vi "PurePursuit.vi"(0 "RobotNeededPathData":T1={"Path"=[], "MaxVel"=0.0, "MaxAccel"=0.0, "Backwards?"=FALSE, "PointSpacing"=0.0, "LookaheadDist"=0.0, "Speed/Curve"=1.8, "SlowDistanceAtEnd"=12.0, "SlowSpeed"=15.0, "MaxDeAccel"=0.0} {"SlowSpeed" format="%#_13g"; "SlowDistanceAtEnd" format="%#_13g"; "Speed/Curve" format="%#_13g"}, 1 "SensorData":T3={"LeftDistance"=0.0, "RightDistance"=0.0, "LeftVelocity"=78.75762159095939, "RightVelocity"=-76.3848555077329, "Angle"=-0.01, "Location"={11.691968699047118, 248.03471515703785}}, 3 "Trackwidth":dbl=40.0 format="%#_13g", 7 "Reset":bool, 14 "Gains":T4={"FFV"=0.0088, "FFA"=0.0017, "Vel PID"={"P"=0.02, "I"=0.0, "D"=0.0}} {"Vel PID"."D" format="%.3f"; "Vel PID"."I" format="%.3f"; "Vel PID"."P" format="%.3f"}) -> (2 "Graph":cluster{cluster{"x":dbl, "y":dbl}[]}[](graph)=[{[{"x"=20.453371592539455, "y"=249.15925394548063}, {"x"=32.451138071473615, "y"=249.2417431099791}, {"x"=44.448056211953954, "y"=249.32366698389004}, {"x"=56.441768980000354, "y"=249.4040828136747}, {"x"=68.42823711154045, "y"=249.48106130123531}, {"x"=80.3987950137465, "y"=249.55036007485356}, {"x"=92.33398719870449, "y"=249.6026243647297}, {"x"=104.19073617112089, "y"=249.61714678939316}, {"x"=115.8737280283298, "y"=249.54805321076083}, {"x"=127.17183717836993, "y"=249.29372430937337}, {"x"=137.61733743281803, "y"=248.62905317811618}, {"x"=146.1740836060984, "y"=247.05537254809167}, {"x"=150.54675993154666, "y"=243.46800813008085}, {"x"=152.39728417160754, "y"=235.46668065740275}, {"x"=152.95934006523578, "y"=225.71717171741398}, {"x"=152.6076327980232, "y"=215.7198087862704}, {"x"=151.107691158904, "y"=206.8096834259849}, {"x"=147.4595538788043, "y"=201.04671193240875}, {"x"=139.23112896790275, "y"=198.5372634006921}, {"x"=128.93601727531555, "y"=197.49649482245655}, {"x"=117.71002861894719, "y"=197.11868334076806}, {"x"=106.06838831868264, "y"=197.04007755842468}, {"x"=94.24922045605804, "y"=197.09639645188625}, {"x"=82.37229762541514, "y"=197.21330877376334}, {"x"=70.51888885096747, "y"=197.35687893558043}, {"x"=58.78593931213765, "y"=197.51094316379152}, {"x"=47.350700340581184, "y"=197.66633376164685}, {"x"=36.58889694113597, "y"=197.8147673041893}, {"x"=27.32521119491603, "y"=197.9433223158581}, {"x"=21.38307030129124, "y"=198.025824964132}]}, {[{"x"=11.691968699047118, "y"=248.03471515703785}, {"x"=23.691968516276667, "y"=248.03680955212963}]}, {[{"x"=152.95934006523578, "y"=225.71717171741398}]}, {[{"x"=26.691968699047116, "y"=248.03471515703785}, {"x"=25.95781644347442, "y"=252.66997007266207}, {"x"=23.827223614671333, "y"=256.85149394142496}, {"x"=20.508747483434213, "y"=260.16997007266207}, {"x"=16.32722361467133, "y"=262.3005629014651}, {"x"=11.69196869904712, "y"=263.03471515703785}, {"x"=7.056713783422908, "y"=262.3005629014651}, {"x"=2.875189914660023, "y"=260.16997007266207}, {"x"=-0.4432862165770928, "y"=256.85149394142496}, {"x"=-2.5738790453801847, "y"=252.66997007266207}, {"x"=-3.308031300952882, "y"=248.03471515703785}, {"x"=-2.5738790453801865, "y"=243.39946024141364}, {"x"=-0.44328621657709455, "y"=239.21793637265077}, {"x"=2.8751899146600195, "y"=235.89946024141364}, {"x"=7.056713783422905, "y"=233.76886741261055}, {"x"=11.691968699047115, "y"=233.03471515703785}, {"x"=16.327223614671325, "y"=233.76886741261055}, {"x"=20.508747483434213, "y"=235.89946024141364}, {"x"=23.82722361467133, "y"=239.21793637265074}, {"x"=25.95781644347442, "y"=243.39946024141364}, {"x"=26.691968699047116, "y"=248.03471515703785}]}, {[{"x"=16.728162111415877, "y"=242.99940064954055}, {"x"=16.48171627411582, "y"=244.55539842807914}, {"x"=15.766502597859695, "y"=245.95908430278035}, {"x"=14.652531180466154, "y"=247.0730557201739}, {"x"=13.248845305764926, "y"=247.78826939643002}, {"x"=11.692847527226334, "y"=248.03471523373008}, {"x"=10.136849748687744, "y"=247.78826939643002}, {"x"=8.733163873986515, "y"=247.0730557201739}, {"x"=7.619192456592972, "y"=245.95908430278035}, {"x"=6.903978780336848, "y"=244.55539842807914}, {"x"=6.6575329430367916, "y"=242.99940064954055}, {"x"=6.903978780336848, "y"=241.44340287100195}, {"x"=7.619192456592971, "y"=240.03971699630074}, {"x"=8.733163873986513, "y"=238.9257455789072}, {"x"=10.136849748687743, "y"=238.21053190265107}, {"x"=11.692847527226332, "y"=237.964086065351}, {"x"=13.248845305764924, "y"=238.21053190265107}, {"x"=14.652531180466152, "y"=238.9257455789072}, {"x"=15.766502597859695, "y"=240.03971699630074}, {"x"=16.48171627411582, "y"=241.44340287100195}, {"x"=16.728162111415877, "y"=242.99940064954055}]}], 4 "LeftValue":dbl=2.7501251582780792, 6 "RightValue":dbl=-2.0461251582780795, 8 "TargetVel":dbl=40.0, 10 "Done":bool)   [LabVIEW 2018]
doc: "Takes in encoder and gyro data, and a path. In real time, calculates the left and right power to send to the motors to travel the path at a specified max speed, acceleration, and lookahead distance"
uses:
  RobotNeededPathData.ctl
panel:
  in  "Max dx/dt":dbl=100.0 format="%#_13g"
  out "TargetVelGraph":dbl(graph)
  out "Waveform Chart":T2(graph)={"l"=198.87785889523798, "dx/dt"=78.75762159095939, "r"=-118.87785889523798, "dx/dt"=-76.3848555077329}
  in  "Average Vels":bool
  # "SET DEFAULTS"
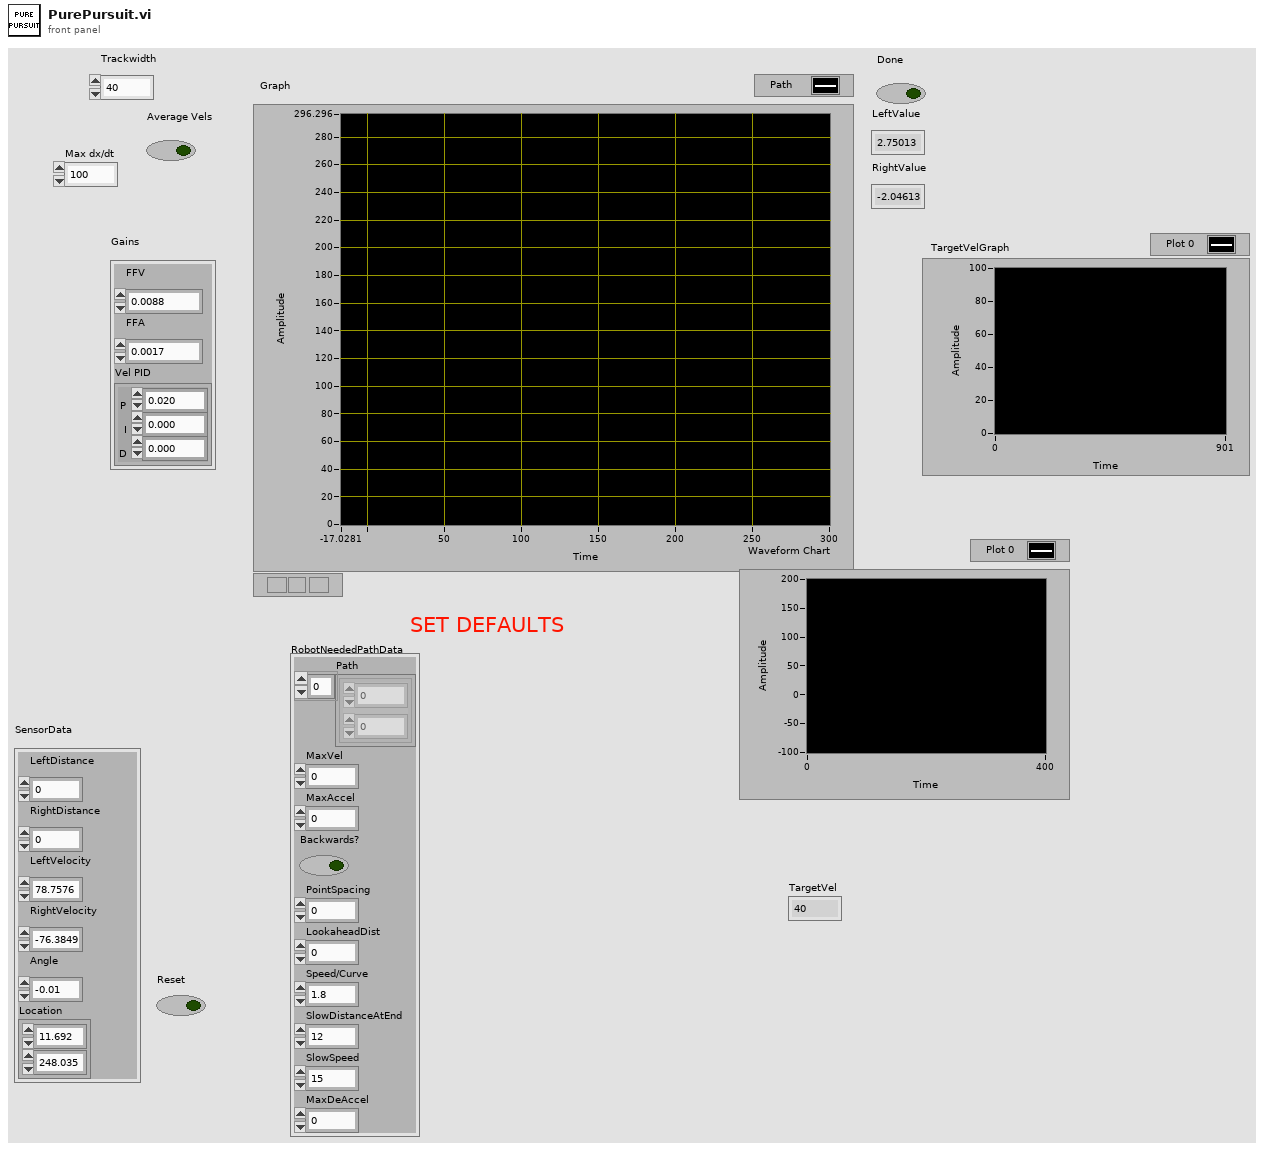
[diagram p1: front panel]
types:
  T1 = typedef "RobotNeededPathData.ctl" = cluster{"Path":cluster{dbl, dbl}[], "MaxVel":dbl, "MaxAccel":dbl, "Backwards?":bool, "PointSpacing":dbl, "LookaheadDist":dbl, "Speed/Curve":dbl, "SlowDistanceAtEnd":dbl, "SlowSpeed":dbl, "MaxDeAccel":dbl}
  T2 = cluster{"l":dbl, "dx/dt":dbl, "r":dbl, "dx/dt":dbl}
  T3 = cluster{"LeftDistance":dbl, "RightDistance":dbl, "LeftVelocity":dbl, "RightVelocity":dbl, "Angle":dbl, "Location":cluster{dbl, dbl}}
  T4 = cluster{"FFV":dbl, "FFA":dbl, "Vel PID":cluster{"P":dbl, "I":dbl, "D":dbl}}
  T5 = cluster{"Path":cluster{"x":dbl, "y":dbl}[], "Spacing":dbl, "DistancesToEnd":dbl[], "Vel":dbl[]}
  T6 = cluster{"Path":cluster{dbl, dbl}[], "PointSpacing":dbl, "DistancesToEnd":dbl[], "Vel":dbl[]}
  T7 = cluster{"l":dbl, "LeftVelocity":dbl, "r":dbl, "RightVelocity":dbl}
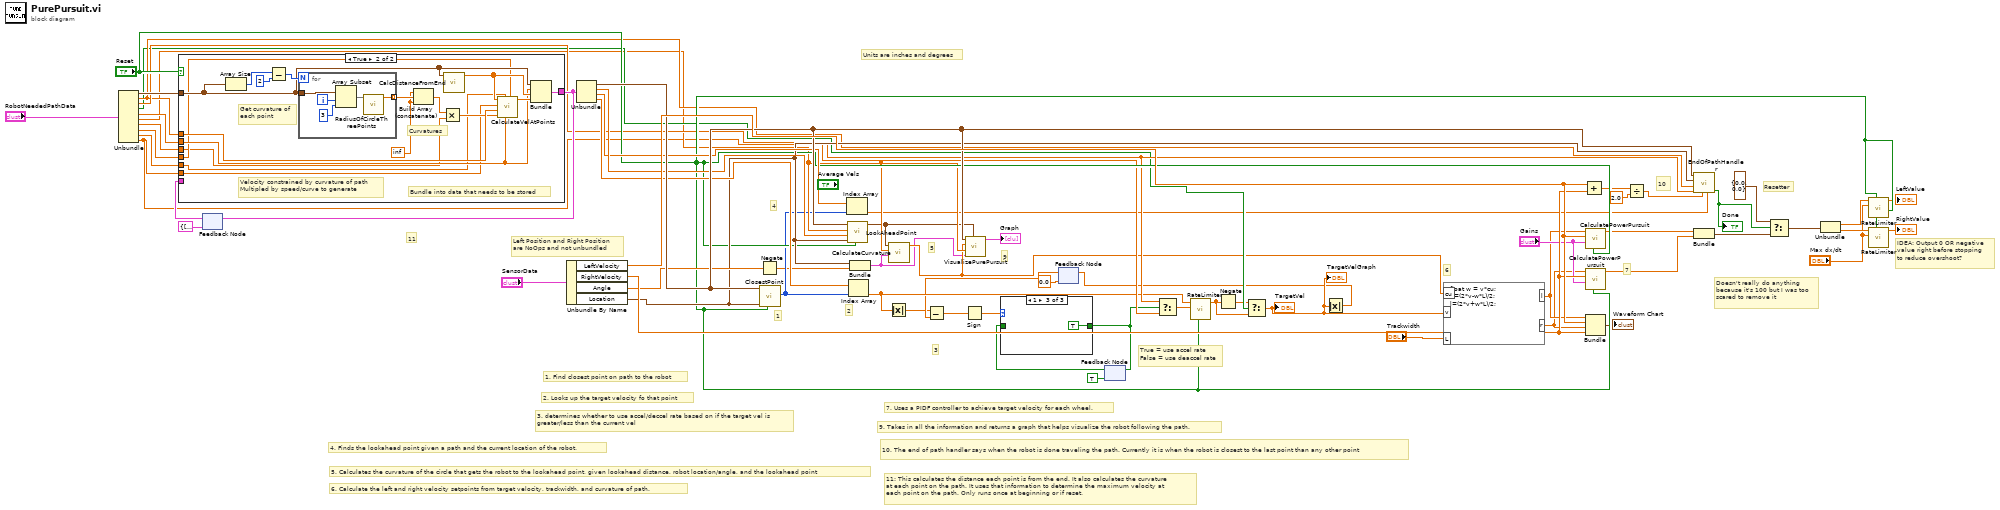
[diagram p0: block diagram]
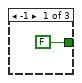
[diagram p2: hidden frame]
diagram:
  # "3"
  # "2"
  # "1"
  # "True = use accel rate\nFalse = use deaccel rate"
  # "Doesn't really do anything\nbecause it's 100 but I was too\nscared to remove it"
  # "IDEA: Output 0 OR negative\nvalue right before stopping\nto reduce overshoot?"
  # "10"
  # "9"
  # "7"
  # "6"
  # "5"
  # "4"
  # "Resetter"
  # "Left Position and Right Position\nare NoOps and not unbundled"
  # "3. determines whether to use accel/deccel rate based on if the target vel is\ngreater/less than the current vel"
  # "2. Looks up the target velocity fo that point"
  # "1. Find closest point on path to the robot"
  # "11: This calculates the distance each point is from the end. It also calculates the curvature\nat each point on the path. It uses that information to determine the maximum velocity at\neach point on the path. Only runs once at beginning or if reset."
  # "11"
  # "10. The end of path handler says when the robot is done traveling the path. Currently it is when the robot is closest to the last point than any other point"
  # "9. Takes in all the information and returns a graph that helps visualize the robot following the path."
  # "7. Uses a PIDF controller to achieve target velocity for each wheel."
  # "6. Calculate the left and right velocity setpoints from target velocity, trackwidth, and curvature of path."
  # "Units are inches and degrees"
  # "5. Calculates the curvature of the circle that gets the robot to the lookahead point, given lookahead distance, robot location/angle, and the lookahead point"
  # "4. Finds the lookahead point given a path and the current location of the robot."
  n1 = Unbundle("RobotNeededPathData") -> ("Path"=w50:cluster{dbl, dbl}[], "MaxVel"=w47:dbl, "MaxAccel"=w48:dbl, "Backwards?"=w46:bool, "PointSpacing"=w49:dbl, "LookaheadDist"=w45:dbl, "Speed/Curve"=w42:dbl, "SlowDistanceAtEnd"=w44:dbl, "SlowSpeed"=w43:dbl, "MaxDeAccel"=w41:dbl)
  n2 = feedback #1(T5 {"Path"=[{"x"=0.0, "y"=0.0}, {"x"=0.0, "y"=46.0}, {"x"=77.25, "y"=97.5}], "Spacing"=0.0, "DistancesToEnd"=[309.52253206522465, 306.5225388483889, 303.52254576348514, 300.5225494135135, 297.5225482930251, 294.5225431892043, 291.52253649479525, 288.5225309404311, 285.52252839669825, 282.52252922985826, 279.52253236801363, 276.5225359199274, 273.5225380077533, 270.5225374640896, 267.5225341651582, 264.5225289486152, 261.52252321975885, 258.52251843460203, 255.52251565052453, 252.52251527415513, 249.52251704698162, 246.52252022727612, 243.52252387624657, 240.5225271449837, 237.52252948071848, 234.5225307115883, 231.5225310121264, 228.5225307841412, 225.52253050297352, 222.52253057724883, 219.522531255923, 216.52253259658312, 213.5225344902357, 210.52253672481638, 207.52253906428678, 204.52254132188853, 201.52254341264756, 198.5225453787386, 195.52254738922483, 192.52254972128023, 189.5225527326013, 186.5225568345679, 183.5225624736694, 180.52257012582595, 177.52258030545136, 174.52259358906986, 171.52261065227918, 168.52263231879937, 165.52265962102405, 162.52269387257934, 159.52273675466557, 156.52279041923995, 153.52285761342083, 150.52294183093122, 147.52304749810799, 144.52318020416902, 141.5233469881785, 138.52355669860665, 135.52382044572104, 132.52415217017628, 129.52456938475245, 126.52509392552396, 123.52575388229783, 120.52658224756205, 117.52762599636499, 114.52893466674816, 111.5305811433295, 108.53265099247815, 105.5352499693053, 102.53851522329074, 99.54261858949184, 96.54777258499563, 93.55424339621041, 90.56236601643654, 87.57255952674781, 84.58534501572932, 81.60137180227034, 78.62143961905741, 75.64655567097594, 72.6779255489502, 69.71706974165639, 66.76578984976493, 63.82625595622302, 60.90103565379168, 57.99306437227732, 55.10557379235981, 52.24189700353533, 49.40502603383819, 46.59675379579783, 43.81612021857386, 41.056705992040605, 38.30212773163372, 35.53590323835957, 32.752089130751756, 29.950811925036337, 27.135602619179224, 24.311917874683846, 21.486403150766286, 18.666614193530503, 15.861028930660632, 13.07925664424869, 10.33239795871144, 7.633538890247935, 4.998382632368401, 2.4460384085185156, 0.0], "Vel"=[309.52253206522465, 306.5225388483889, 303.52254576348514, 300.5225494135135, 297.5225482930251, 294.5225431892043, 291.52253649479525, 288.5225309404311, 285.52252839669825, 282.52252922985826, 279.52253236801363, 276.5225359199274, 273.5225380077533, 270.5225374640896, 267.5225341651582, 264.5225289486152, 261.52252321975885, 258.52251843460203, 255.52251565052453, 252.52251527415513, 249.52251704698162, 246.52252022727612, 243.52252387624657, 240.5225271449837, 237.52252948071848, 234.5225307115883, 231.5225310121264, 228.5225307841412, 225.52253050297352, 222.52253057724883, 219.522531255923, 216.52253259658312, 213.5225344902357, 210.52253672481638, 207.52253906428678, 204.52254132188853, 201.52254341264756, 198.5225453787386, 195.52254738922483, 192.52254972128023, 189.5225527326013, 186.5225568345679, 183.5225624736694, 180.52257012582595, 177.52258030545136, 174.52259358906986, 171.52261065227918, 168.52263231879937, 165.52265962102405, 162.52269387257934, 159.52273675466557, 156.52279041923995, 153.52285761342083, 150.52294183093122, 147.52304749810799, 144.52318020416902, 141.5233469881785, 138.52355669860665, 135.52382044572104, 132.52415217017628, 129.52456938475245, 126.52509392552396, 123.52575388229783, 120.52658224756205, 117.52762599636499, 114.52893466674816, 111.5305811433295, 108.53265099247815, 105.5352499693053, 102.53851522329074, 99.54261858949184, 96.54777258499563, 93.55424339621041, 90.56236601643654, 87.57255952674781, 84.58534501572932, 81.60137180227034, 78.62143961905741, 75.64655567097594, 72.6779255489502, 69.71706974165639, 66.76578984976493, 63.82625595622302, 60.90103565379168, 57.99306437227732, 55.10557379235981, 52.24189700353533, 49.40502603383819, 46.59675379579783, 43.81612021857386, 41.056705992040605, 38.30212773163372, 35.53590323835957, 32.752089130751756, 29.950811925036337, 27.135602619179224, 24.311917874683846, 21.486403150766286, 18.666614193530503, 15.861028930660632, 13.07925664424869, 10.33239795871144, 7.633538890247935, 4.998382632368401, 2.4460384085185156, 0.0]} ("PathData")) -> (w54:T5)
  n3 = case shown="True" "Reset" {
    tunnel: [w65 w81] -> w53
    tunnel: w54 -> [w65 _]
    tunnel: w47 -> [_ w72]
    tunnel: w50 -> [_ w74]
    tunnel: w49 -> [_ w70]
    tunnel: w44 -> [_ w69]
    tunnel: w43 -> [_ w68]
    tunnel: w42 -> [_ w67]
    tunnel: w41 -> [_ w66]
    frame False {
    }
    frame True {
      w76 = inf
      # "Velocity constrained by curvature of path\nMultipled by speed/curve to generate"
      # "Bundle into data that needs to be stored"
      # "Get curvature of\neach point"
      # "Curvatures"
      n4 = Array Size(array=w74) -> (size(s)=w77:i32)
      n5 = Subtract(x=w77, y=2) -> (x-y=w78:i32)
      n6 = for {
        N: w78 -> [_]
        tunnel: w74 -> [w87]
        tunnel: [w83] -> w79 mode=indexing
        i -> [w86]
        n7 = Array Subset(array=w87, index=w86, length=3) -> (w84:cluster{dbl, dbl}[])
        n8 = call "RadiusOfCircleThreePoints.vi"("Points"=w84) -> ("R"=w83:dbl)  [unwired: 10 in]
      }
      n9 = Build Array (concatenate)(w76, w79, w76) -> (w80:dbl[])
      n10 = Multiply(x=w80, y=w67) -> (x*y=w71:dbl[])
      n11 = call "CalcDistanceFromEnd.vi"("Path"=w74) -> ("DistancesToEnd"=w73:dbl[])  [unwired: 10 in]
      n12 = call "CalculateVelAtPoints.vi"("DistanceSlowAtEnd"=w69, "Spacing"=w70, "SlowSpeed"=w68, "MaxVels"=w71, "MaxVel"=w72, "MaxAccel"=w66, "DistancesToEnd"=w73) -> ("Vel"=w82:dbl[])  [unwired: 4 in]
      n13 = Bundle("Path"=w74, "PointSpacing"=w70, "DistancesToEnd"=w73, "Vel"=w82) -> (w81:T6)  [unwired: 1 in]
    }
  }
  n14 = feedback-in #1(w53) -> ()
  n15 = Unbundle By Name("SensorData") -> ("LeftVelocity"=w63:dbl, "RightVelocity"=w62:dbl, "Angle"=w57:dbl, "Location"=w56:cluster{dbl, dbl})
  n16 = Unbundle(w53) -> ("Path"=w61:cluster{"x":dbl, "y":dbl}[], "PointSpacing"=w60:dbl, "DistancesToEnd"=w59:dbl[], "Vel"=w58:dbl[])
  n17 = Negate(x=w57) -> (-x=w21:dbl)
  n18 = call "ClosestPoint.vi"("Reset"="Reset", "Robot"=w56, "Path"=w61) -> ("ClosestIndex"=w25:i32)  [unwired: 7 in, 1 out]
  n19 = Index Array(array=w59, index=w25) -> (element=w26:dbl)
  n20 = call "LookAheadPoint.vi"("Reset"="Reset", "Robot"=w56, "Spacing"=w60, "LookAhead"=w45, "Path"=w61) -> ("Point"=w36:cluster{"x":dbl, "y":dbl})  [unwired: 5 in, 1 out]
  n21 = Index Array(array=w58, index=w25) -> (element=w6:dbl)
  n22 = Bundle("Location"=w56, w21) -> (w37:cluster{"Location":cluster{dbl, dbl}, dbl})  [unwired: 1 in]
  n23 = Absolute Value(x=w6) -> (abs(x)=w2:dbl)
  n24 = call "CalculateCurvature.vi"("Robot"=w37, "Lookahead"=w45, "Point"=w36) -> ("Curvature"=w38:dbl)  [unwired: 8 in]
  n25 = call "VisualizePurePursuit.vi"("Lookahead Point"=w36, "Robot"=w37, "Lookahead"=w45, "Curvature"=w38, "Path"=w61) -> ("Graph"=→"Graph":cluster{cluster{"x":dbl, "y":dbl}[]}[])  [unwired: 6 in]
  n26 = feedback #2(0.0) -> (w3:dbl)
  n27 = Subtract(x=w2, y=w3) -> (x-y=w12:dbl)
  n28 = Sign(1:w12) -> (0:w11:dbl)
  n29 = feedback #3(TRUE) -> (w10:bool)
  n30 = case shown="1" w11 {
    tunnel: [FALSE w89 TRUE] -> w8
    tunnel: w10 -> [_ w89 _]
    frame -1 {
    }
    frame 0, Default {
    }
    frame 1 {
    }
  }
  n31 = feedback-in #3(w8) -> ()
  n32 = Select(t=w48, s=w8, f=w41) -> (s? t:f=w7:dbl)
  n33 = call "RateLimiter.vi"("Reset"="Reset", "Max dx/dt"=w7, "Input"=w6) -> ("Output"=w14:dbl)  [unwired: 8 in]
  n34 = Negate(x=w14) -> (-x=w13:dbl)
  n35 = Select(t=w13, s=w46, f=w14) -> (s? t:f=w5:dbl)
  "TargetVel" <- w5
  "TargetVelGraph" <- w5
  n36 = Absolute Value(x=w5) -> (abs(x)=w4:dbl)
  n37 = feedback-in #2(w4) -> ()
  n38 = formula code="float w = v*cu;\nr =(2*v-w*L)/2;\nl=(2*v+w*L)/2;"("L"="Trackwidth", "cu"=w38, "v"=w5) -> ("r"=w28:dbl, "l"=w30:dbl)
  n39 = Add(x=w63, y=w62) -> (x+y=w33:dbl)
  n40 = call "CalculatePowerPursuit.vi"("Reset"="Reset", "Gains"="Gains", "Vel"=w63, "Target Vel"=w30) -> ("Power"=w35:dbl)  [unwired: 7 in]
  n41 = call "CalculatePowerPursuit.vi"("Reset"="Reset", "Gains"="Gains", "Vel"=w62, "Target Vel"=w28) -> ("Power"=w34:dbl)  [unwired: 7 in]
  n42 = Bundle("l"=w30, "LeftVelocity"=w63, "r"=w28, "RightVelocity"=w62) -> (→"Waveform Chart":T7)  [unwired: 1 in]
  n43 = Divide(x=w33, y=2.0) -> (x/y=w31:dbl)
  n44 = call "EndOfPathHandler.vi"("DistanceToEnd"=w26, "CurrentVel"=w31, "MaxAccel"=w48, "MaxVel"=w47, "RobotLocation"=w56, "Path"=w61) -> ("Done"=w20:bool)  [unwired: 2 in, 3 out]
  "Done" <- w20
  n45 = Bundle("Power"=w35, "Power"=w34) -> (w24:cluster{"Power":dbl, "Power":dbl})  [unwired: 1 in]
  n46 = Select(t=cluster{"Power":dbl, "Power":dbl} {"Power"=0.0, "Power"=0.0}, s=w20, f=w24) -> (s? t:f=w22:cluster{"Power":dbl, "Power":dbl})
  n47 = Unbundle(w22) -> ("Power"=w19:dbl, "Power"=w18:dbl)
  n48 = call "RateLimiter.vi"("Reset"="Reset", "Max dx/dt"="Max dx/dt", "Input"=w19) -> ("Output"=→"LeftValue":dbl)  [unwired: 8 in]
  n49 = call "RateLimiter.vi"("Reset"="Reset", "Max dx/dt"="Max dx/dt", "Input"=w18) -> ("Output"=→"RightValue":dbl)  [unwired: 8 in]
